vi "returnTDMSinfo.vi"(1 "error in (no error)":errorcluster, 2 "Refnum in":refnum<k34>) -> (0 "TDMS contents":cluster{string, string[]}[](array[cluster]))   [LabVIEW 2013]
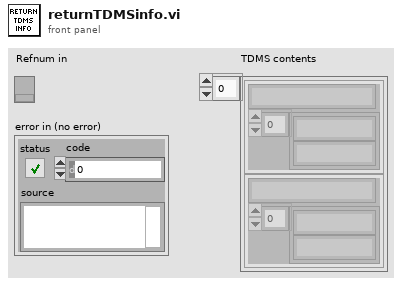
[diagram p1: front panel]
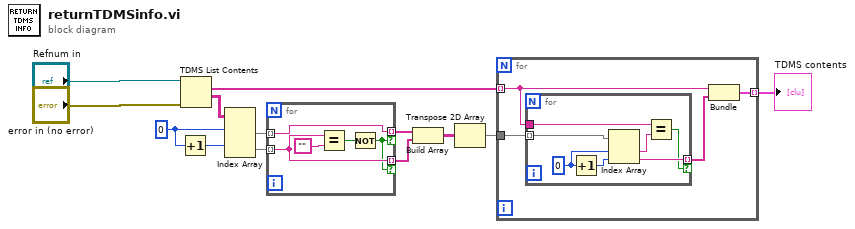
[diagram p0: block diagram]
diagram:
  w4 = 0
  n1 = Increment(x=w4) -> (x+1=w6:i32)
  n2 = TDMS List Contents(4:"error in (no error)", 7:"Refnum in") -> (1:w3:string[][], 2:w10:string[])  [unwired: 1 in, 2 out]
  n3 = Index Array(array=w3, index (row) #1=w4, index (row) #2=w6) -> (element #1=w5:string[], element #2=w7:string[])  [unwired: 2 in]
  n4 = for {
    tunnel: w5 -> [w18] mode=indexing
    tunnel: w7 -> [w17] mode=indexing
    tunnel: [w18] -> w8 mode=indexing if=w14
    tunnel: [w17] -> w9 mode=indexing if=w14
    n5 = Equal?(x=w17, y="") -> (x = y?=w15:bool)
    n6 = Not(x=w15) -> (.not. x?=w14:bool)
  }
  n7 = Build Array(w8, w9) -> (w11:string[][])
  n8 = Transpose 2D Array(2D array=w11) -> (transposed array=w12:string[][])
  n9 = for {
    tunnel: w10 -> [w20] mode=indexing
    tunnel: w12 -> [w22]
    tunnel: [w19] -> w13 mode=indexing
    n10 = for {
      tunnel: w20 -> [w29]
      tunnel: w22 -> [w28] mode=indexing
      tunnel: [w24] -> w21 mode=indexing if=w23
      w26 = 0
      n11 = Increment(x=w26) -> (x+1=w27:i32)
      n12 = Index Array(array=w28, index #1=w26, index #2=w27) -> (element #1=w25:string, element #2=w24:string)
      n13 = Equal?(x=w29, y=w25) -> (x = y?=w23:bool)
    }
    n14 = Bundle(w20, w21) -> (w19:cluster{string, string[]})  [unwired: 1 in]
  }
  "TDMS contents" <- w13
